vi "string to slave diagnostics.vi"(8 "error in":errorcluster, 11 "data string":string) -> (0 "error out":errorcluster, 3 "slave diagnostics":T1[](array[typedef]))   [LabVIEW 2013, in "Profibus Module configuration.lvclass"]
uses:
  Profibus Module configuration.lvclass
  slave diagnostic configuration.ctl
  <vilib>/NI/Tag Bus Module Framework/channel/TBM channel.lvclass
  error throw specification.ctl
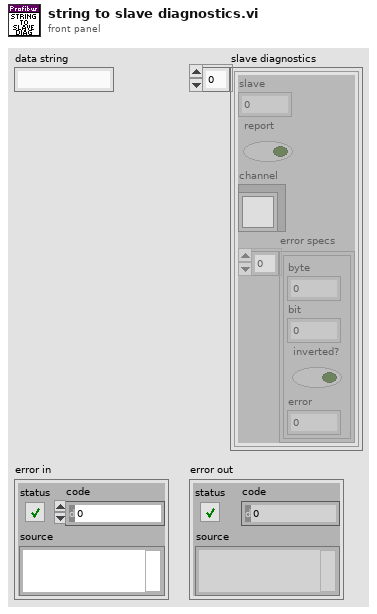
[diagram p1: front panel]
types:
  T1 = typedef "Profibus Module configuration.lvclass/slave diagnostic configuration.ctl" = cluster{"slave":i8, "report":bool, "channel":refnum<class "TBM channel.lvclass">, "error specs":T2[]}
  T2 = typedef "Profibus Module configuration.lvclass/error throw specification.ctl" = cluster{"byte":i32, "bit":i32, "inverted?":bool, "error":i32}
  T3 = cluster{"slave":i8, "identifier":string, "channel data":string, "error specs":T2[]}[]
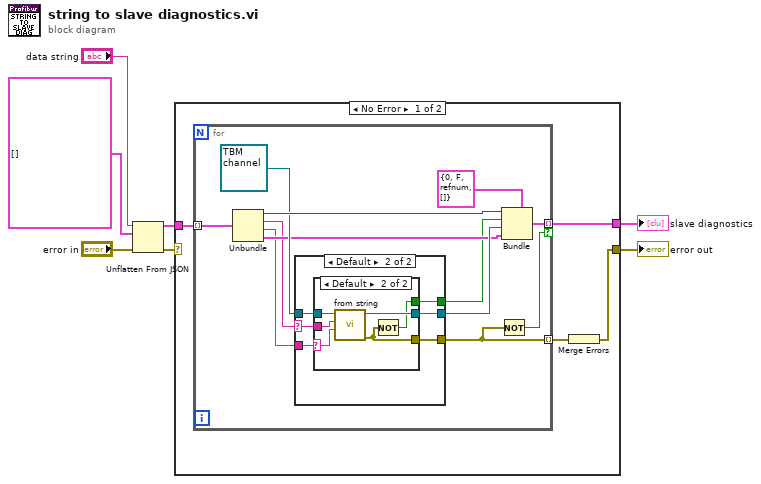
[diagram p0: block diagram]
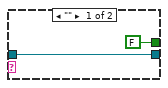
[diagram p2: hidden frame]
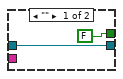
[diagram p3: hidden frame]
diagram:
  n1 = Unflatten From JSON(JSON string="data string", type and defaults=T3 [], error in (no error)="error in") -> (value=w3:T3, error out=w5:errorcluster)  [unwired: 4 in]
  n2 = case shown="No Error" w5 {
    selector: w5 -> [_ w40]
    tunnel: [w11 w40] -> w4
    tunnel: w3 -> [w9 _]
    tunnel: [w10 _] -> w2
    frame No Error {
      n3 = for {
        tunnel: [w22] -> w10 mode=indexing if=w21
        tunnel: w9 -> [w20] mode=indexing
        tunnel: [w16] -> w8 mode=indexing
        n4 = Unbundle(w20) -> ("slave"=w19:i8, "identifier"=w14:string, "channel data"=w12:string, "error specs"=w15:T2[])
        n5 = case shown="Default" w14 {
          selector: w14 -> [_ w26]
          tunnel: refnum<class "TBM channel.lvclass"> refnum ("channel in") -> [w25 w31]
          tunnel: [w25 w30] -> w17
          tunnel: [_ w29] -> w16
          tunnel: [FALSE w27] -> w13
          tunnel: w12 -> [_ w28]
          frame "" {
          }
          frame Default {
            n6 = case shown="Default" w28 {
              selector: w28 -> [_ w34]
              tunnel: w31 -> [w33 w39]
              tunnel: [w33 w38] -> w30
              tunnel: [_ w37] -> w29
              tunnel: [FALSE w36] -> w27
              tunnel: w26 -> [_ w35]
              frame "" {
              }
              frame Default {
                n7 = call-dynamic "from string.vi"("channel data"=w34, "identifier"=w35, "channel in"=w39) -> ("error out"=w37:errorcluster, "channel out"=w38:refnum<class "TBM channel.lvclass">)  [unwired: 7 in]
                n8 = Not(x=w37) -> (.not. x?=w36:bool)
              }
            }
          }
        }
        n9 = Not(x=w16) -> (.not. x?=w21:bool)
        n10 = Bundle(cluster=T1 {"slave"=0, "report"=FALSE, "channel"=refnum, "error specs"=[]} ("diagnostics settings"), "slave"=w19, "report"=w13, "channel"=w17, "error specs"=w15) -> (w22:T1)
      }
      n11 = Merge Errors(w8) -> (w11:errorcluster)
    }
    frame Error {
    }
  }
  "slave diagnostics" <- w2
  "error out" <- w4
